vi "PlotTve.vi"(7 "Clear? (f)":bool, 8 "error in (no error)":errorcluster, 11 "Data real time":dbl[](array[numeric])) -> (0 "error out":errorcluster, 3 "TVE":dbl[][](graph))   [LabVIEW 2018, in "Visualization.lvlib"]
uses:
  Visualization.lvlib
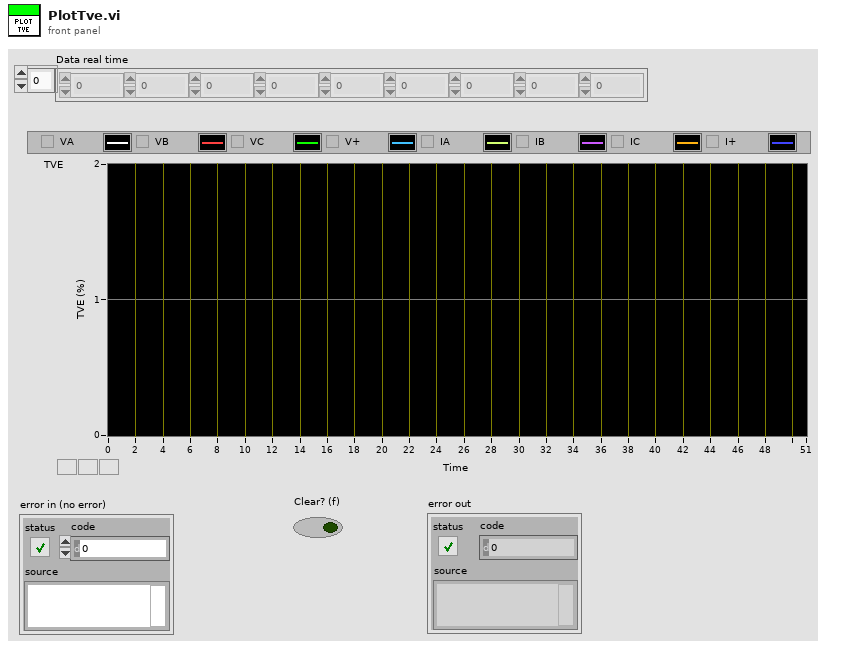
[diagram p1: front panel]
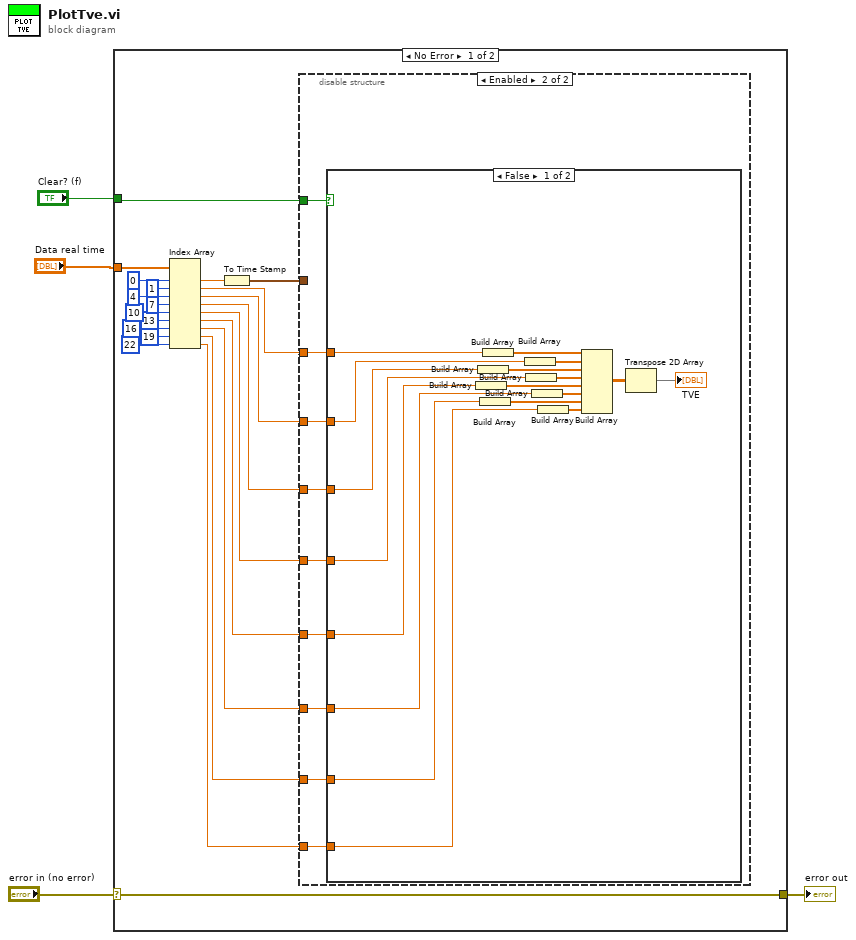
[diagram p0: block diagram]
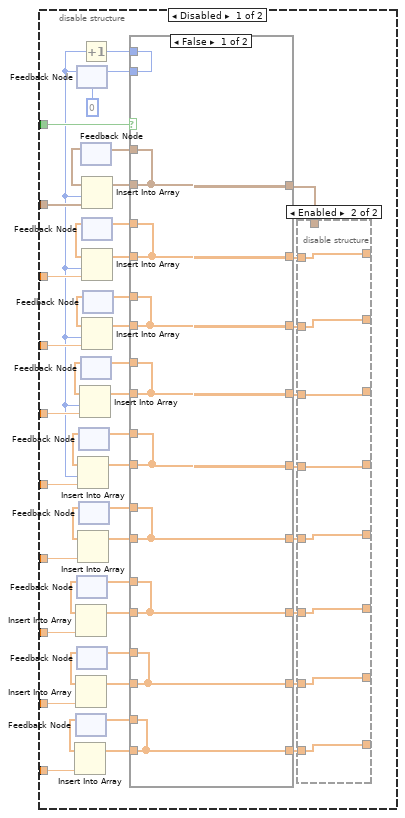
[diagram p2: hidden frame]
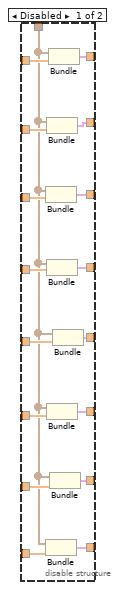
[diagram p3: hidden frame]
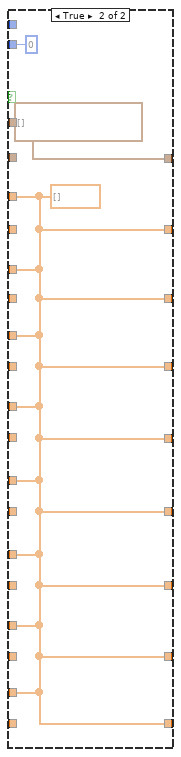
[diagram p4: hidden frame]
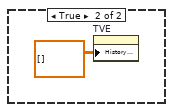
[diagram p5: hidden frame]
diagram:
  n1 = case shown="No Error" "error in (no error)" {
    selector: "error in (no error)" -> [w13 w151]
    tunnel: "Clear? (f)" -> [w26 _]
    tunnel: "Data real time" -> [w25 _]
    tunnel: [w13 w151] -> w1
    frame No Error {
      n2 = Index Array(array=w25, index #1=0 ("index"), index #2=1 ("index"), index #3=4 ("index"), index #4=7 ("index"), index #5=10 ("index"), index #6=13 ("index"), index #7=16 ("index"), index #8=19 ("index"), index #9=22 ("index")) -> (element #1=w19:dbl, element #2=w23:dbl, element #3=w22:dbl, element #4=w21:dbl, element #5=w20:dbl, element #6=w9:dbl, element #7=w8:dbl, element #8=w7:dbl, element #9=w5:dbl)
      n3 = To Time Stamp(1:w19) -> (0:w24:timestamp)
      n4 = disable-structure shown="Enabled" {
        disable-tunnel: w26 -> [w84 w131]
        disable-tunnel: w24 -> [w83 _]
        disable-tunnel: w23 -> [w82 w130]
        disable-tunnel: w22 -> [w81 w129]
        disable-tunnel: w21 -> [w80 w128]
        disable-tunnel: w20 -> [w79 w127]
        disable-tunnel: w9 -> [w49 w126]
        disable-tunnel: w8 -> [w48 w125]
        disable-tunnel: w7 -> [w47 w124]
        disable-tunnel: w5 -> [w33 w123]
        frame Disabled {
          n5 = feedback #1() -> (w27:dbl[])  [unwired: 1 in]
          n6 = Insert Into Array(array=w27, new element=w33) -> (w32:dbl[])  [unwired: 1 in]
          n7 = feedback #2(u32 0) -> (w74:u32)
          n8 = feedback #3() -> (w35:dbl[])  [unwired: 1 in]
          n9 = Insert Into Array(array=w35, new element=w48) -> (w46:dbl[])  [unwired: 1 in]
          n10 = feedback #4() -> (w34:dbl[])  [unwired: 1 in]
          n11 = Insert Into Array(array=w34, new element=w47) -> (w45:dbl[])  [unwired: 1 in]
          n12 = feedback #5() -> (w73:dbl[])  [unwired: 1 in]
          n13 = Insert Into Array(array=w73, index=w74, new element=w79) -> (w71:dbl[])
          n14 = feedback #6() -> (w36:dbl[])  [unwired: 1 in]
          n15 = Insert Into Array(array=w36, new element=w49) -> (w51:dbl[])  [unwired: 1 in]
          n16 = Increment(x=w74) -> (x+1=w60:u32)
          n17 = feedback #7() -> (w56:timestamp[])  [unwired: 1 in]
          n18 = feedback #8() -> (w70:dbl[])  [unwired: 1 in]
          n19 = Insert Into Array(array=w70, index=w74, new element=w80) -> (w68:dbl[])
          n20 = Insert Into Array(array=w56, index=w74, new element=w83) -> (w57:timestamp[])
          n21 = feedback #9() -> (w64:dbl[])  [unwired: 1 in]
          n22 = Insert Into Array(array=w64, index=w74, new element=w82) -> (w62:dbl[])
          n23 = feedback #10() -> (w67:dbl[])  [unwired: 1 in]
          n24 = Insert Into Array(array=w67, index=w74, new element=w81) -> (w65:dbl[])
          n25 = case shown="False" w84 {
            tunnel: w57 -> [w118 _]
            tunnel: [w118 w121] -> w58
            tunnel: w60 -> [w119 _]
            tunnel: [w119 u32 0] -> w61
            tunnel: [w118 w121] -> w30
            tunnel: w62 -> [w117 _]
            tunnel: [w117 w120] -> w63
            tunnel: [w117 w120] -> w78
            tunnel: w65 -> [w116 _]
            tunnel: [w116 w120] -> w66
            tunnel: [w116 w120] -> w77
            tunnel: w68 -> [w115 _]
            tunnel: [w115 w120] -> w69
            tunnel: w71 -> [w114 _]
            tunnel: [w114 w120] -> w72
            tunnel: [w115 w120] -> w76
            tunnel: [w114 w120] -> w75
            tunnel: w51 -> [w113 _]
            tunnel: [w113 w120] -> w50
            tunnel: [w112 w120] -> w44
            tunnel: w46 -> [w112 _]
            tunnel: [w111 w120] -> w43
            tunnel: w45 -> [w111 _]
            tunnel: [w113 w120] -> w39
            tunnel: [w112 w120] -> w38
            tunnel: [w111 w120] -> w37
            tunnel: [w110 w120] -> w31
            tunnel: w32 -> [w110 _]
            tunnel: [w110 w120] -> w28
            frame False {
            }
            frame True {
              w120 = dbl[] []
              w121 = timestamp[] []
            }
          }
          n26 = feedback-in #1(w28) -> ()
          n27 = feedback-in #2(w61) -> ()
          n28 = feedback-in #3(w38) -> ()
          n29 = feedback-in #4(w37) -> ()
          n30 = feedback-in #5(w72) -> ()
          n31 = feedback-in #6(w39) -> ()
          n32 = feedback-in #7(w58) -> ()
          n33 = feedback-in #8(w69) -> ()
          n34 = feedback-in #9(w63) -> ()
          n35 = feedback-in #10(w66) -> ()
          n36 = disable-structure shown="Enabled" {
            disable-tunnel: w78 -> [w101 w109]
            disable-tunnel: w77 -> [w100 w108]
            disable-tunnel: w76 -> [w99 w107]
            disable-tunnel: w75 -> [w98 w106]
            disable-tunnel: [w97 w109] -> w55
            disable-tunnel: [w96 w108] -> w54
            disable-tunnel: [w95 w107] -> w53
            disable-tunnel: [w94 w106] -> w52
            disable-tunnel: w50 -> [w93 w105]
            disable-tunnel: w44 -> [w92 w104]
            disable-tunnel: w43 -> [w91 w103]
            disable-tunnel: [w90 w105] -> w42
            disable-tunnel: [w89 w104] -> w41
            disable-tunnel: [w88 w103] -> w40
            disable-tunnel: w31 -> [w87 w102]
            disable-tunnel: w30 -> [w86 _]
            disable-tunnel: [w85 w102] -> w29
            frame Disabled {
              n37 = Bundle(w86, w99) -> (w95:cluster{timestamp[], dbl[]})  [unwired: 1 in]
              n38 = Bundle(w86, w87) -> (w85:cluster{timestamp[], dbl[]})  [unwired: 1 in]
              n39 = Bundle(w86, w100) -> (w96:cluster{timestamp[], dbl[]})  [unwired: 1 in]
              n40 = Bundle(w86, w98) -> (w94:cluster{timestamp[], dbl[]})  [unwired: 1 in]
              n41 = Bundle(w86, w92) -> (w89:cluster{timestamp[], dbl[]})  [unwired: 1 in]
              n42 = Bundle(w86, w101) -> (w97:cluster{timestamp[], dbl[]})  [unwired: 1 in]
              n43 = Bundle(w86, w91) -> (w88:cluster{timestamp[], dbl[]})  [unwired: 1 in]
              n44 = Bundle(w86, w93) -> (w90:cluster{timestamp[], dbl[]})  [unwired: 1 in]
            }
            frame Enabled {
            }
          }
        }
        frame Enabled {
          n45 = case shown="False" w131 {
            tunnel: w130 -> [w149 _]
            tunnel: w129 -> [w148 _]
            tunnel: w128 -> [w147 _]
            tunnel: w127 -> [w146 _]
            tunnel: w126 -> [w145 _]
            tunnel: w125 -> [w144 _]
            tunnel: w124 -> [w143 _]
            tunnel: w123 -> [w142 _]
            frame False {
              n46 = Build Array(w145) -> (w136:dbl[])
              n47 = Build Array(w147) -> (w138:dbl[])
              n48 = Build Array(w143) -> (w134:dbl[])
              n49 = Build Array(w149) -> (w140:dbl[])
              n50 = Build Array(w148) -> (w139:dbl[])
              n51 = Build Array(w146) -> (w137:dbl[])
              n52 = Build Array(w144) -> (w135:dbl[])
              n53 = Build Array(w142) -> (w133:dbl[])
              n54 = Build Array(w140, w139, w138, w137, w136, w135, w134, w133) -> (w141:dbl[][])
              n55 = Transpose 2D Array(2D array=w141) -> (transposed array=→"TVE":dbl[][])
            }
            frame True {
              n56 = property on="TVE" class="WFChart (strict)"("History Data"=dbl[][] []) -> ()  [unwired: 2 in, 2 out]
            }
          }
        }
      }
    }
    frame Error {
    }
  }
  "error out" <- w1
